vi "Set Gate Mode.vi"(8 "error in (no error)":errorcluster, 11 "gatemode":i32) -> (0 "error out":errorcluster, 3 "function return":u32)   [LabVIEW 2014, in "atmcd32d.lvlib"]
doc: "unsigned int WINAPI SetGateMode(int gatemode);"
uses:
  atmcd32d.lvlib
  atmcd32d.dll
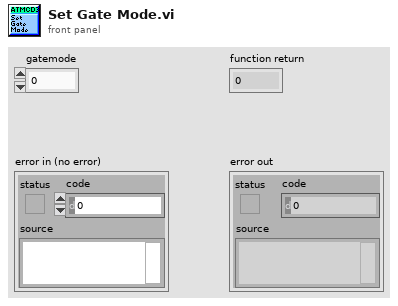
[diagram p1: front panel]
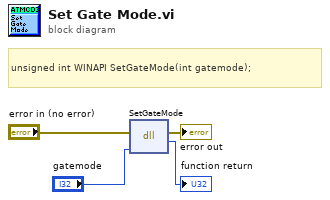
[diagram p0: block diagram]
diagram:
  # "unsigned int WINAPI SetGateMode(int gatemode);"
  n1 = dll-call lib="C:/Users/Bakir/Documents/Lambda2-Testing/lib/Andorlib/atmcd32d.*" fn="SetGateMode"(error in="error in (no error)", "gatemode"="gatemode") -> (error out=→"error out":errorcluster, →"function return":u32)  [unwired: 3 in, 1 out]
